vi "Read Test Data (AC Phase C Manual Mode).vi"(0 "VISA resource name":refnum<visa-resource-name>, 11 "error in (no error)":errorcluster) -> (4 "VISA resource name out":refnum<visa-resource-name>, 6 "Test Meter Data Output":T1 {"Power Apparent (VA)" format="%.1f"; "Crest Factor" format="%.2f"; "Power Resistive (VAR)" format="%.3f"; "Frequency (Hz)" format="%.1f"; "Voltage (V)" format="%.1f"; "RMS Current (A)" format="%.3f"; "Power (W)" format="%.1f"; "Peak Current (A)" format="%.1f"; "Power Factor" format="%.1f"}, 15 "error out":errorcluster)   [LabVIEW 2016, in "APT 300XAC Series.lvlib"]
doc: "Reads the Manual mode <B>active data being displayed on the LCD display</B> while the test is in process. It also gives the last data taken when the test sequence compled. \n\nIn Manual Mode the output data cluster has the following data.\n\n1. Memory\n2. Timer (s)\n3. Frequency (Hz)\n4. Voltage (V)\n5. RMS Current (A)\n6. Peak Current (A)\n7. Power (W)\n8. Power Factor\n9. Status"
uses:
  APT 300XAC Series.lvlib
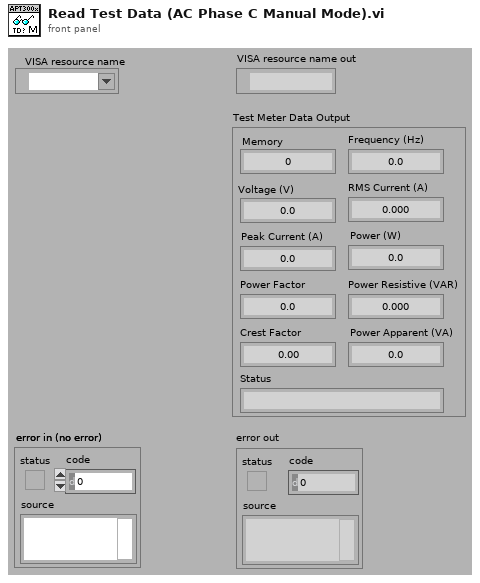
[diagram p1: front panel]
types:
  T1 = cluster{"Memory":dbl, "Frequency (Hz)":dbl, "Voltage (V)":dbl, "RMS Current (A)":dbl, "Peak Current (A)":dbl, "Power (W)":dbl, "Power Factor":dbl, "Status":string, "Power Resistive (VAR)":dbl, "Crest Factor":dbl, "Power Apparent (VA)":dbl}
  T2 = cluster{"Memory":i32, "Frequency":dbl, "Volt":dbl, "Current":dbl, "Peak Current":dbl, "Power":dbl, "Power Factor":dbl, "Status":string, "Power Resistive":dbl, "Crest Factor":dbl, "Power Apparent":dbl}
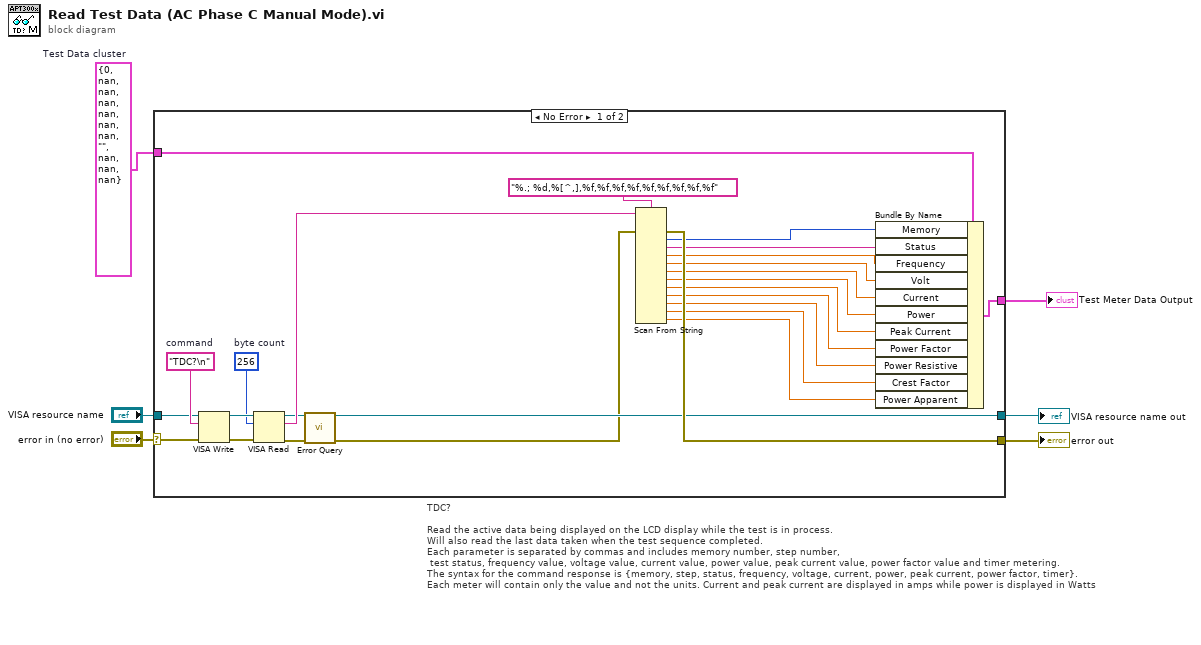
[diagram p0: block diagram]
diagram:
  w2 = T2 {"Memory"=0, "Frequency"=nan, "Volt"=nan, "Current"=nan, "Peak Current"=nan, "Power"=nan, "Power Factor"=nan, "Status"="", "Power Resistive"=nan, "Crest Factor"=nan, "Power Apparent"=nan}  # Test Data cluster
  # "TDC?\n\nRead the active data being displayed on the LCD display while the test is in process. \nWill also read the last data taken when the test sequence completed. \nEach parameter is separated by commas and includes memory number, step number,\n test status, frequency value, voltage value, current value, power value, peak current value, power factor value and timer metering. \nThe syntax for the command response is {memory, step, status, frequency, voltage, current, power, peak current, power factor, timer}. \nEach meter will contain only the value and not the units. Current and peak current are displayed in amps while power is displayed in Watts"
  n1 = case shown="No Error" "error in (no error)" {
    selector: "error in (no error)" -> [w25 w34]
    tunnel: "VISA resource name" -> [w26 w35]
    tunnel: [w11 w35] -> w4
    tunnel: [w24 w34] -> w3
    tunnel: [w29 w33] -> w1
    tunnel: w2 -> [w28 w33]
    frame No Error {
      w27 = "TDC?\n"  # command
      w30 = u32 256  # byte count
      n2 = VISA Write(VISA resource name=w26, write buffer=w27, error in (no error)=w25) -> (VISA resource name out=w32:refnum<visa-resource-name>, error out=w31:errorcluster)  [unwired: 1 out]
      n3 = VISA Read(VISA resource name=w32, byte count=w30, error in (no error)=w31) -> (VISA resource name out=w22:refnum<visa-resource-name>, read buffer=w23:string, error out=w21:errorcluster)  [unwired: 1 out]
      n4 = call "Error Query.vi"("VISA resource name"=w22, "error in (no error)"=w21) -> ("VISA resource name out"=w11:refnum<visa-resource-name>, "error out"=w10:errorcluster)  [unwired: 10 in, 2 out]
      n5 = Scan From String(format string="%.; %d,%[^,],%f,%f,%f,%f,%f,%f,%f,%f,%f", input string=w23, error in=w10) -> (error out=w24:errorcluster, output 1=w19:i32, output 2=w18:string, output 3=w17:dbl, output 4=w16:dbl, output 5=w15:dbl, output 6=w14:dbl, output 7=w13:dbl, output 8=w12:dbl, output 9=w9:dbl, output 10=w8:dbl, output 11=w7:dbl)  [unwired: 12 in, 2 out]
      n6 = Bundle By Name(cluster=w28, "Memory"=w19, "Status"=w18, "Frequency"=w17, "Volt"=w16, "Current"=w15, "Power"=w14, "Peak Current"=w13, "Power Factor"=w12, "Power Resistive"=w9, "Crest Factor"=w8, "Power Apparent"=w7) -> (w29:T2)
    }
    frame Error {
    }
  }
  "VISA resource name out" <- w4
  "error out" <- w3
  "Test Meter Data Output" <- w1
